vi "IMGInfo.vi"(8 "Error in":errorcluster caption="Error in (no error)", 11 "ImgPath":path) -> (0 "Error out":errorcluster, 1 "Landscape":bool, 2 "image size (pixels)":cluster{"x":i16, "y":i16}, 3 "ImgPath out":path, 4 "error":bool)   [LabVIEW 2016, in "EPUB.lvclass"]
uses:
  EPUB.lvclass
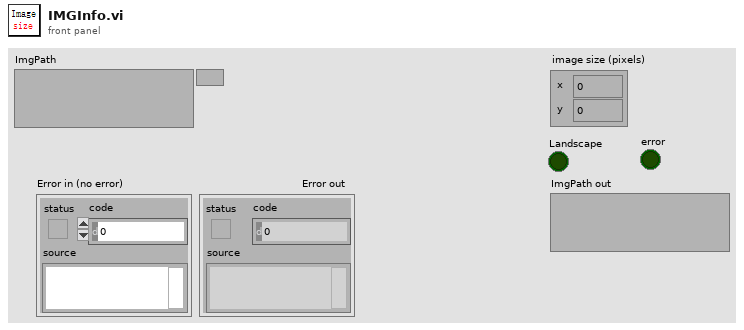
[diagram p1: front panel]
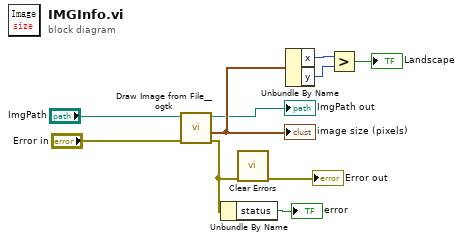
[diagram p0: block diagram]
diagram:
  n1 = call <userlib>:"Draw Image from File__ogtk.vi"("error in (no error)"="Error in", "path to image file"="ImgPath") -> ("error out"=w3:errorcluster, "image size (pixels)"=w9:cluster{"x":i16, "y":i16}, "dup path"=→"ImgPath out":path)  [unwired: 6 in, 1 out]
  "image size (pixels)" <- w9
  n2 = Unbundle By Name(w3) -> ("status"=→"error":bool)
  n3 = call <vilib>:"Clear Errors.vi"("error in (no error)"=w3) -> ("error out"=→"Error out":errorcluster)  [unwired: 5 in, 1 out]
  n4 = Unbundle By Name(w9) -> ("x"=w8:i16, "y"=w7:i16)
  n5 = Greater?(x=w8, y=w7) -> (0:→"Landscape":bool)
